vi "Determine if the NOK in A row Counter needs to be increased and remember new NOK tests.vi"(9 "NOK tests from previous DUT":string[](array[string]), 11 "Current Failure set":string[](array[string])) -> (1 "Increase NOK Three In A Row VCounter":bool, 3 "New NOK test from previous DUT":string[](array[string]))   [LabVIEW 2023, in "In a row NOK.lvlib"]
uses:
  In a row NOK.lvlib
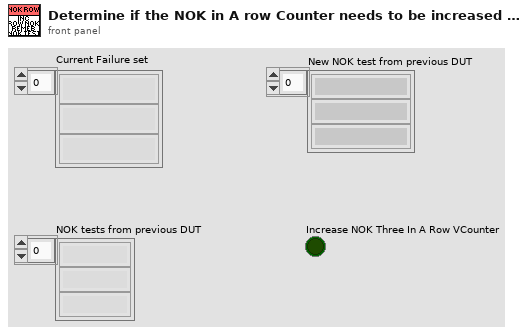
[diagram p1: front panel]
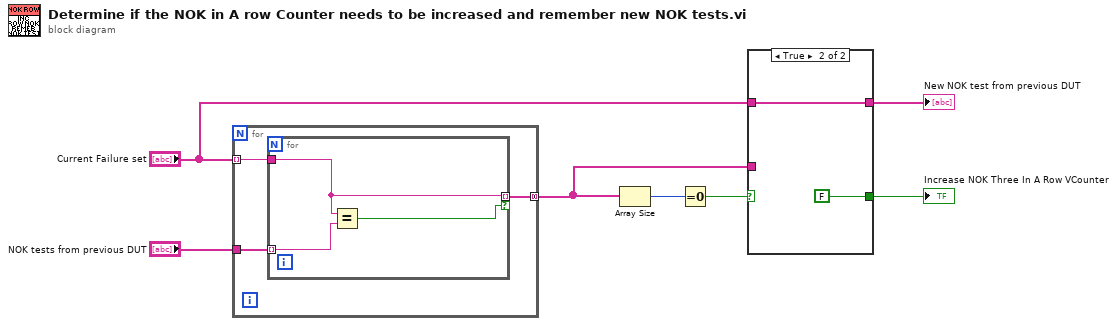
[diagram p0: block diagram]
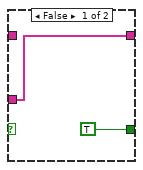
[diagram p2: hidden frame]
diagram:
  n1 = for {
    tunnel: "Current Failure set" -> [w9] mode=indexing
    tunnel: "NOK tests from previous DUT" -> [w10]
    tunnel: [w8] -> w3 mode=concatenating
    n2 = for {
      tunnel: w10 -> [w13] mode=indexing
      tunnel: w9 -> [w12]
      tunnel: [w12] -> w8 mode=indexing if=w11
      n3 = Equal?(x=w12, y=w13) -> (x = y?=w11:bool)
    }
  }
  n4 = Array Size(array=w3) -> (size(s)=w6:i32)
  n5 = Equal To 0?(x=w6) -> (x = 0?=w5:bool)
  n6 = case shown="True" w5 {
    tunnel: "Current Failure set" -> [_ w17]
    tunnel: w3 -> [w15 _]
    tunnel: [w15 w17] -> w2
    tunnel: [TRUE FALSE] -> w1
    frame False {
    }
    frame True {
    }
  }
  "New NOK test from previous DUT" <- w2
  "Increase NOK Three In A Row VCounter" <- w1
